vi "Benchmark.vi"() -> ()   [LabVIEW 2012]
doc: "This example uses an assembly-level call to obtain precise timestamps from RT targets. The purpose of this example is to gather timing information on a user's VI by running it for several iterations. The example obtains several consecutive 64-bit timestamps, which are stored in an array and used later to produce a histogram of execution time. This VI can self-calibrate by subtracting out the overhead of calling NI Get Timestamp.vi from the array of timing data.\n\nINSTRUCTIONS:\n1. Select a number of iterations and warmup iterations to exclude from the benchmark.\n2. Use calibration if you want to exclude the overhead of the timestamping operation.\n3. Go to the diagram and insert the code you want to benchmark."
uses:
  <vilib>/NI_Real-Time Target Support.lvlib
panel:
  out "index of element":i32
  in  "element":u8
  in  "unsigned 8bit integer":u8[](array[numeric])
  out "mean time (uS)":dbl format="%.2f"
  in  "Warmup iterations":i32=10
  in  "Calibrate?":bool
  out "execution histogram":T1(graph)
  out "execution times (uS)":dbl[](graph)
  out "max jitter (uS)":dbl format="%.2f"
  out "standard deviation (uS)":dbl format="%.2f"
  in  "Iterations":i32=1000
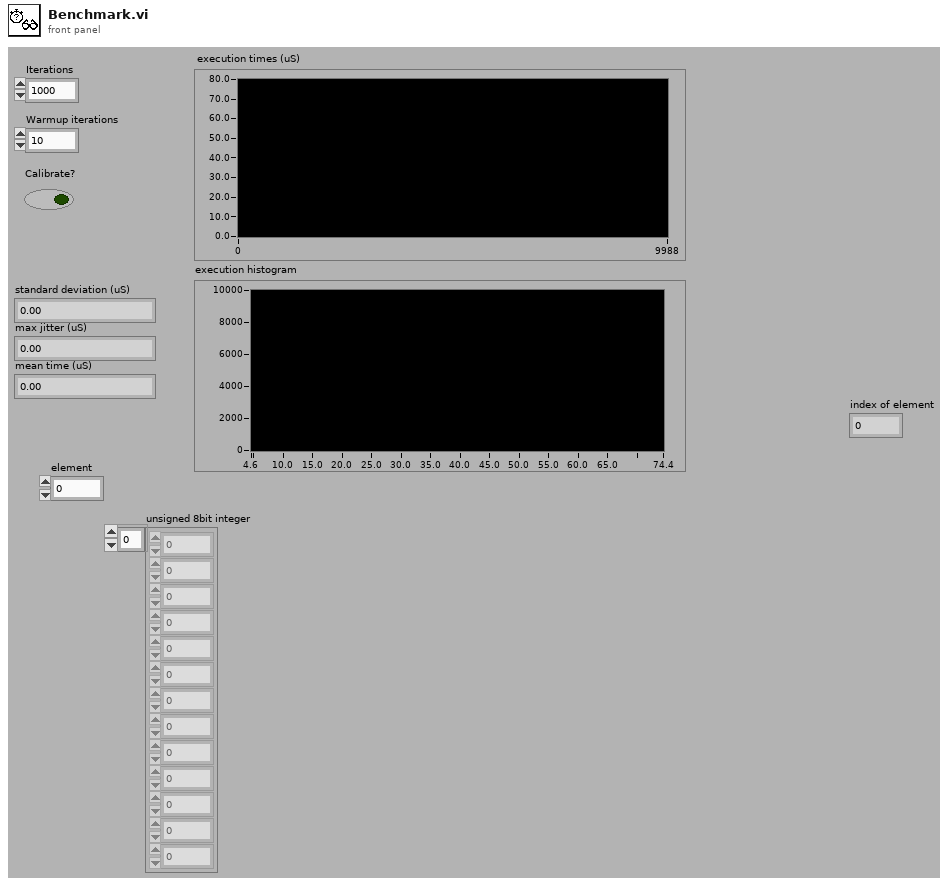
[diagram p1: front panel]
types:
  T1 = cluster{"X Values":dbl[], "Histogram: h(x)":i32[]}
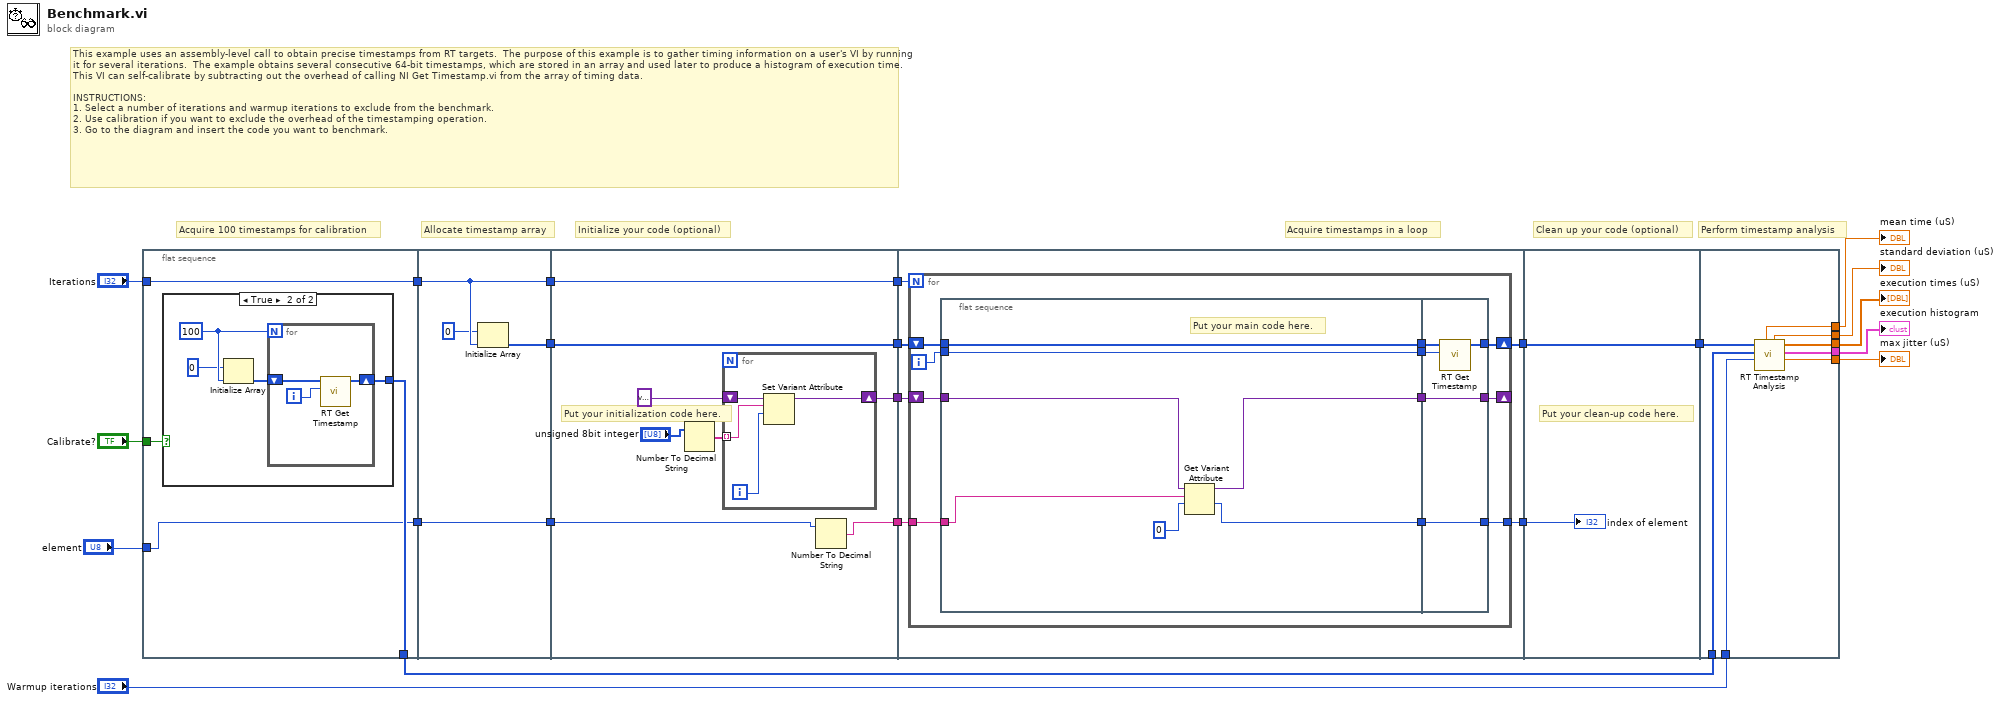
[diagram p0: block diagram]
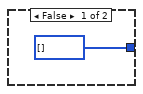
[diagram p2: hidden frame]
diagram:
  # "This example uses an assembly-level call to obtain precise timestamps from RT targets.  The purpose of this example is to gather timing information on a user's VI by running it for several iterations.  The example obtains several consecutive 64-bit timestamps, which are stored in an array and used later to produce a histogram of execution time. This VI can self-calibrate by subtracting out the overhead of calling NI Get Timestamp.vi from the array of timing data.\n\nINSTRUCTIONS:\n1. Select a number of iterations and warmup iterations to exclude from the benchmark.\n2. Use calibration if you want to exclude the overhead of the timestamping operation.\n3. Go to the diagram and insert the code you want to benchmark."
  # "Perform timestamp analysis"
  # "Acquire timestamps in a loop"
  # "Clean up your code (optional)"
  # "Initialize your code (optional)"
  # "Allocate timestamp array"
  # "Acquire 100 timestamps for calibration"
  n1 = flat-sequence {
    tunnel: "Iterations" -> [w26]
    tunnel: [w26] -> w16
    tunnel: "Calibrate?" -> [w25]
    tunnel: [w24] -> w13
    tunnel: "element" -> [w23]
    tunnel: [w23] -> w3
    tunnel: [w37] -> w18
    tunnel: [w38] -> w17
    tunnel: w16 -> [w37]
    tunnel: [w35] -> w4
    tunnel: w3 -> [w35]
    tunnel: [w46] -> w20
    tunnel: [w45] -> w19
    tunnel: w18 -> [w46]
    tunnel: w17 -> [w45]
    tunnel: [w39] -> w5
    tunnel: w4 -> [w40]
    tunnel: [w41] -> w1
    tunnel: [w56] -> w21
    tunnel: w20 -> [w55]
    tunnel: w19 -> [w54]
    tunnel: w5 -> [w53]
    tunnel: [w52] -> w2
    tunnel: w1 -> [w51]
    tunnel: w21 -> [w81]
    tunnel: [w81] -> w14
    tunnel: w2 -> [w80]
    tunnel: w14 -> [w89]
    tunnel: w13 -> [w88]
    tunnel: [w87] -> w11
    tunnel: [w86] -> w10
    tunnel: [w85] -> w9
    tunnel: [w84] -> w12
    tunnel: "Warmup iterations" -> [w83]
    tunnel: [w82] -> w7
    frame #0 {
      n2 = case shown="True" w25 {
        tunnel: [u64[] [] w31] -> w24
        frame False {
        }
        frame True {
          w29 = 100
          n3 = Initialize Array(u64 0, w29) -> (w30:u64[])
          n4 = for {
            N: w29 -> [_]
            shift-right: [w32] -> w31
            shift-left: w30 -> [w33]
            i -> [w34]
            n5 = call <vilib>:"RT Get Timestamp.vi"("iteration"=w34, "timestamp array in"=w33) -> ("timestamp array out"=w32:u64[])  [unwired: 1 in, 8 out]
          }
        }
      }
    }
    frame #1 {
      n6 = Initialize Array(u64 0, w37) -> (w38:u64[])
    }
    frame #2 {
      # "Put your initialization code here."
      n7 = Number To Decimal String(number="unsigned 8bit integer") -> (decimal integer string=w44:string[])  [unwired: 1 in]
      n8 = for {
        tunnel: w44 -> [w49] mode=indexing
        shift-right: [w47] -> w41
        shift-left: variant ("variant") -> [w50]
        i -> [w48]
        n9 = Set Variant Attribute(Variant=w50, name=w49, value=w48) -> (Variant out=w47:variant)  [unwired: 1 in, 2 out]
      }
      n10 = Number To Decimal String(number=w40) -> (decimal integer string=w39:string)  [unwired: 1 in]
    }
    frame #3 {
      n11 = for {
        N: w55 -> [_]
        shift-right: [w67] -> w56
        shift-left: w54 -> [w66]
        tunnel: w53 -> [w62]
        tunnel: [w60] -> w52
        shift-right: [w57] -> _
        shift-left: w51 -> [w59]
        i -> [w65]
        n12 = flat-sequence {
          tunnel: w66 -> [w74]
          tunnel: [w74] -> w64
          tunnel: w65 -> [w73]
          tunnel: [w73] -> w63
          tunnel: w62 -> [w68]
          tunnel: [w69] -> w61
          tunnel: w59 -> [w72]
          tunnel: [w70] -> w58
          tunnel: [w79] -> w67
          tunnel: w64 -> [w77]
          tunnel: w63 -> [w78]
          tunnel: w61 -> [w76]
          tunnel: [w76] -> w60
          tunnel: w58 -> [w75]
          tunnel: [w75] -> w57
          frame #0 {
            # "Put your main code here."
            n13 = Get Variant Attribute(Variant=w72, name=w68, default value (empty Variant)=0 ("index of element")) -> (duplicate Variant=w70:variant, value=w69:i32)  [unwired: 1 in, 2 out]
          }
          frame #1 {
            n14 = call <vilib>:"RT Get Timestamp.vi"("iteration"=w78, "timestamp array in"=w77) -> ("timestamp array out"=w79:u64[])  [unwired: 1 in, 8 out]
          }
        }
      }
    }
    frame #4 {
      # "Put your clean-up code here."
      "index of element" <- w80
    }
    frame #5 {
      n15 = call <vilib>:"RT Timestamp Analysis.vi"("warmup iterations"=w83, "calibration array"=w88, "timestamp array"=w89) -> ("max jitter (uS)"=w86:dbl, "execution histogram"=w87:T1, "execution times (uS)"=w84:dbl[], "standard deviation (uS)"=w85:dbl, "mean time (uS)"=w82:dbl)  [unwired: 1 in, 3 out]
    }
  }
  "execution times (uS)" <- w12
  "max jitter (uS)" <- w10
  "standard deviation (uS)" <- w9
  "execution histogram" <- w11
  "mean time (uS)" <- w7
